vi "Open URL in Default Browser (string).vi"(4 "error in (no error)":errorcluster, 7 "URL":string) -> (0 "error out":errorcluster, 3 "URL out":string)   [LabVIEW 2017]
doc: "Displays a URL or HTML file in the default Web browser. If the URL or path you wire to this VI contains a space character, the VI encodes the space as %20 before displaying the URL or HTML file in the Web browser. Wire data to the <B>URL</B> input to determine the polymorphic instance to use or manually select the instance."
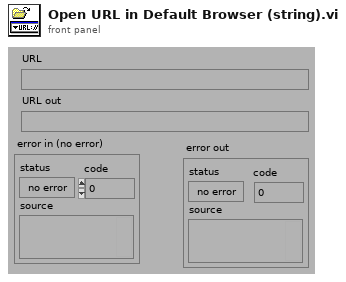
[diagram p1: front panel]
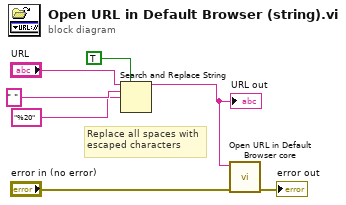
[diagram p0: block diagram]
diagram:
  # "Replace all spaces with\nescaped characters"
  n1 = Search and Replace String(replace all?=TRUE ("replace all? (F)"), input string="URL", search string=" ", replace string="%20" ("replace string (\"\")")) -> (result string=w3:string)  [unwired: 4 in, 3 out]
  "URL out" <- w3
  n2 = call "Open URL in Default Browser core.vi"("error in (no error)"="error in (no error)", "url"=w3) -> ("error out"=→"error out":errorcluster)  [unwired: 4 in, 1 out]
